vi "RT Get Root Path.vi"() -> (3 "Root Path out":path)   [LabVIEW 2015]
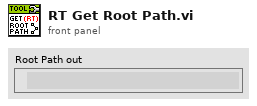
[diagram p1: front panel]
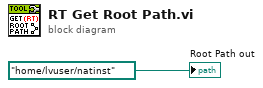
[diagram p0: block diagram]
diagram:
  "Root Path out" <- path "/home/lvuser/natinst" ("Cfg File Root Path")
